vi "SetText.vi"(8 "error in (no error)":errorcluster, 10 "Text":string, 11 "Markdown in":refnum<class "Markdown.lvclass">) -> (0 "error out":errorcluster, 3 "Markdown out":refnum<class "Markdown.lvclass">)   [LabVIEW 2021, in "Markdown.lvlib" / "Markdown.lvclass"]
uses:
  Markdown.lvclass
  Markdown.lvclass/Markdown.ctl
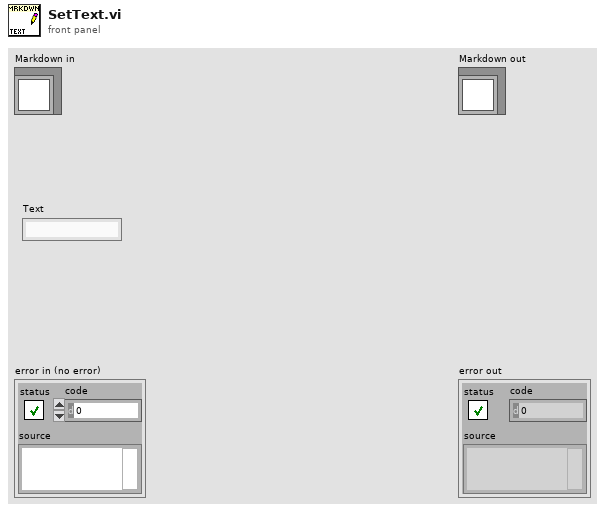
[diagram p1: front panel]
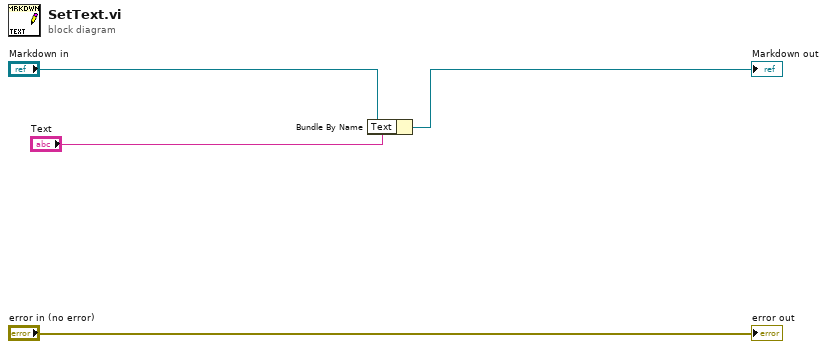
[diagram p0: block diagram]
diagram:
  n1 = Bundle By Name(cluster="Markdown in", "Text"="Text") -> (→"Markdown out":refnum<class "Markdown.lvclass">)
  "error out" <- "error in (no error)"
